vi "Contents Summary Text.vi"(11 "Message":refnum<class "VarMessage.lvclass">) -> (2 "Contents Summary Text":string, 3 "Message":refnum<class "VarMessage.lvclass">)   [LabVIEW 2011, in "Messenging.lvlib" / "VarMessage.lvclass"]
uses:
  VarMessage.lvclass
  <userlib>/_OpenG.lib/lvdata/lvdata.llb/Type Descriptor Enumeration__ogtk.ctl
  Send/Send.lvclass
  TextVarientMessage/MSG.lvclass
panel:
  out "Varient":variant
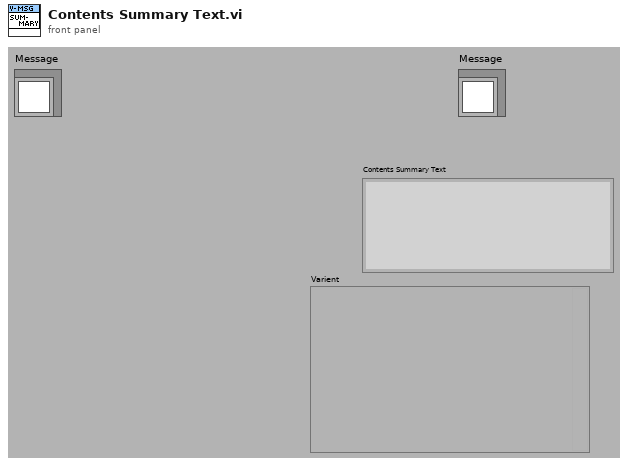
[diagram p1: front panel]
types:
  T1 = typedef "Type Descriptor Enumeration__ogtk.ctl" = enum8{"<Null>", "I8", "I16", "I32", "I64", "U8", "U16", "U32", "U64", "SGL", "DBL", "EXT", "CSG", "CDB", "CXT", "0x0F", "0x10", "0x11", "0x12", "0x13", "0x14", "Enum U8", "Enum U16", "Enum U32", "Enum U64", "SGL PQ", "DBL PQ", "EXT PQ", "CSG PQ", "CDB PQ", "CXT PQ", "0x1F", "0x20", "Boolean", "0x22", "0x23", "0x24", "0x25", "0x26", "0x27", "0x28", "0x29", "0x2A", "0x2B", "0x2C", "0x2D", "0x2E", "0x2F", "String", "0x31", "Path", "Pict", "0x34", "0x35", "0x36", "DAQ", "0x38", "0x39", "0x3A", "0x3B", "0x3C", "0x3D", "0x3E", "0x3F", "Array", "0x41", "0x42", "0x43", "0x44", "0x45", "0x46", "0x47", "0x48", "0x49", "0x4A", "0x4B", "0x4C", "0x4D", "0x4E", "0x4F", "Cluster", "0x51", "0x52", "Variant", "Waveform", "0x55", "0x56", "0x57", "0x58", "0x59", "0x5A", "0x5B", "0x5C", "0x5D", "0x5E", "0x5F", "0x60", "0x61", "0x62", "0x63", "0x64", "0x65", "0x66", "0x67", "0x68", "0x69", "0x6A", "0x6B", "0x6C", "0x6D", "0x6E", "0x6F", "Refnum"}
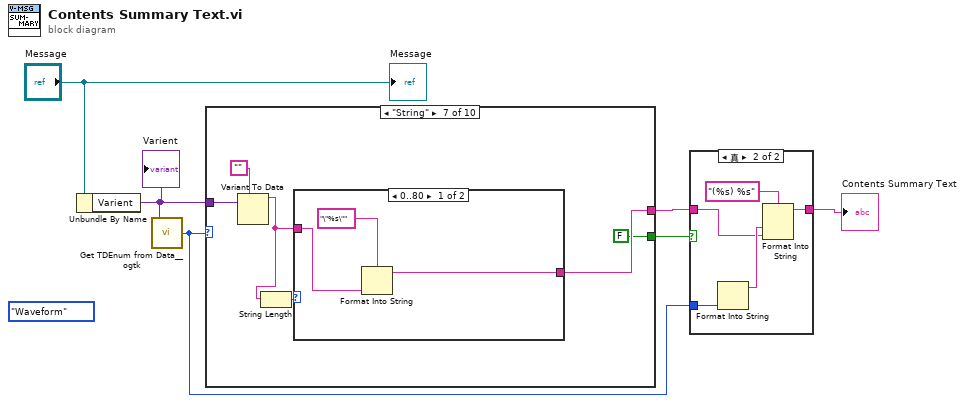
[diagram p0: block diagram]
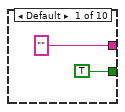
[diagram p3: hidden frame]
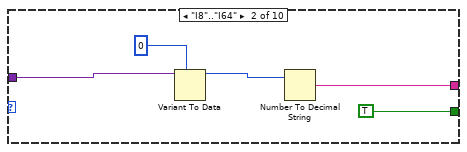
[diagram p4: hidden frame]
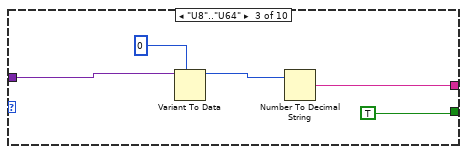
[diagram p5: hidden frame]
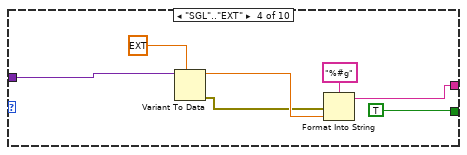
[diagram p6: hidden frame]
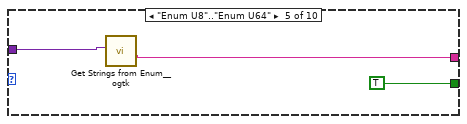
[diagram p7: hidden frame]
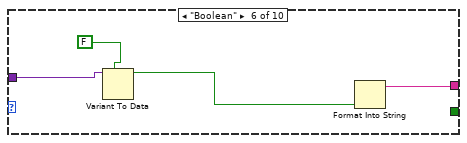
[diagram p8: hidden frame]
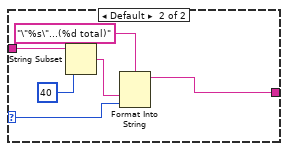
[diagram p9: hidden frame]
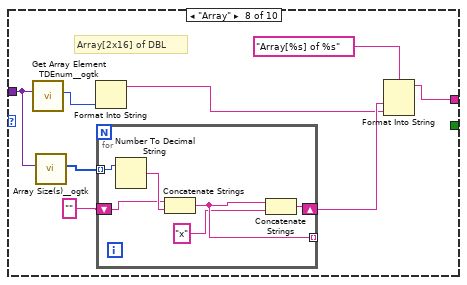
[diagram p10: hidden frame]
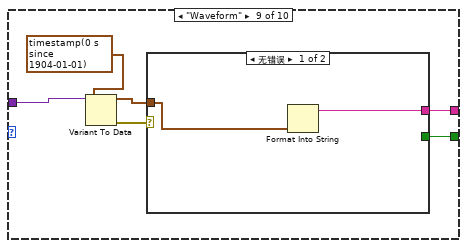
[diagram p11: hidden frame]
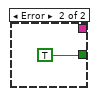
[diagram p12: hidden frame]
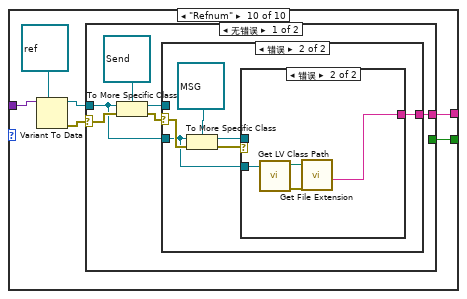
[diagram p13: hidden frame]
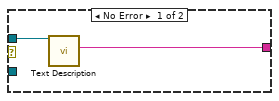
[diagram p14: hidden frame]
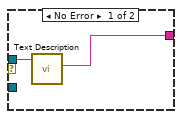
[diagram p15: hidden frame]
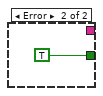
[diagram p16: hidden frame]
diagram:
  (unwired) Type_Descriptor_Enumeration__ogtk."Waveform" ("Type Descriptor Enumeration")
  n1 = Unbundle By Name("Message") -> ("Varient"=w1:variant)
  "Varient" <- w1
  n2 = call <userlib>:"Get TDEnum from Data__ogtk.vi"("Data"=w1) -> ("Type Descriptor Enumeration"=w5:T1)  [unwired: 4 out]
  n3 = case shown="\"String\"" w5 {
    tunnel: w1 -> [_ w13 w18 w25 w28 w31 w38 w54 w67 w76]
    tunnel: ["" w10 w15 w20 w26 w32 w34 w50 w63 w72] -> w3
    tunnel: [TRUE TRUE TRUE TRUE TRUE _ FALSE _ w62 w71] -> w2
    frame Default {
    }
    frame "I8".."I64" {
      n4 = Variant To Data(type=i64 0, Variant=w13) -> (data=w11:i64)  [unwired: 1 in, 1 out]
      n5 = Number To Decimal String(number=w11) -> (decimal integer string=w10:string)  [unwired: 1 out]
    }
    frame "U8".."U64" {
      n6 = Variant To Data(type=u64 0, Variant=w18) -> (data=w16:u64)  [unwired: 1 in, 1 out]
      n7 = Number To Decimal String(number=w16) -> (decimal integer string=w15:string)  [unwired: 1 out]
    }
    frame "SGL".."EXT" {
      n8 = Variant To Data(type=ext 0.0, Variant=w25) -> (data=w23:ext, error out=w22:errorcluster)  [unwired: 1 in]
      n9 = Format Into String(format string="%#g", error in=w22, w23) -> (resulting string=w20:string)  [unwired: 1 in, 1 out]
    }
    frame "Enum U8".."Enum U64" {
      n10 = call <userlib>:"Get Strings from Enum__ogtk.vi"("Enum"=w28) -> ("String Value"=w26:string)  [unwired: 1 in, 9 out]
    }
    frame "Boolean" {
      n11 = Variant To Data(type=FALSE, Variant=w31) -> (data=w29:bool)  [unwired: 1 in, 1 out]
      n12 = Format Into String(w29) -> (resulting string=w32:string)  [unwired: 3 in, 1 out]
    }
    frame "String" {
      n13 = Variant To Data(type="", Variant=w38) -> (data=w35:string)  [unwired: 1 in, 1 out]
      n14 = String Length(string=w35) -> (length=w36:i32)
      n15 = case shown="0..80" w36 {
        selector: w36 -> [_ w44]
        tunnel: w35 -> [w40 w47]
        tunnel: [w41 w43] -> w34
        frame 0..80 {
          n16 = Format Into String(format string="\"%s\"", w40) -> (resulting string=w41:string)  [unwired: 2 in, 1 out]
        }
        frame Default {
          n17 = String Subset(string=w47, length (rest)=40 ("length (rest)")) -> (substring=w42:string)  [unwired: 1 out]
          n18 = Format Into String(format string="\"%s\"...(%d total)", w42, w44) -> (resulting string=w43:string)  [unwired: 2 in, 1 out]
        }
      }
    }
    frame "Array" {
      # "Array[2x16] of DBL"
      n19 = call <userlib>:"Get Array Element TDEnum__ogtk.vi"("Array"=w54) -> ("Element Type"=w55:T1)  [unwired: 1 in, 9 out]
      n20 = call <userlib>:"Array Size(s)__ogtk.vi"("Array"=w54) -> ("Size(s)"=w53:u32[])  [unwired: 1 in, 9 out]
      n21 = Format Into String(w55) -> (resulting string=w48:string)  [unwired: 3 in, 1 out]
      n22 = for {
        tunnel: w53 -> [w61] mode=indexing
        shift-right: [w58] -> w49
        shift-left: "" -> [w59]
        tunnel: [w57] -> _ mode=indexing
        n23 = Number To Decimal String(number=w61) -> (decimal integer string=w60:string)  [unwired: 1 out]
        n24 = Concatenate Strings(w59, w60) -> (w57:string)
        n25 = Concatenate Strings(w57, "x") -> (w58:string)
      }
      n26 = Format Into String(format string="Array[%s] of %s", w49, w48) -> (resulting string=w50:string)  [unwired: 2 in, 1 out]
    }
    frame "Waveform" {
      n27 = Variant To Data(type=timestamp(0 s since 1904-01-01), Variant=w67) -> (data=w64:timestamp, error out=w65:errorcluster)  [unwired: 1 in]
      n28 = case shown="无错误" w65 {
        tunnel: w64 -> [w69 _]
        tunnel: [w68 _] -> w63
        tunnel: [_ TRUE] -> w62
        frame No Error {
          n29 = Format Into String(w69) -> (resulting string=w68:string)  [unwired: 3 in, 1 out]
        }
        frame Error {
        }
      }
    }
    frame "Refnum" {
      n30 = Variant To Data(type=refnum<class> refnum ("LabVIEW Object"), Variant=w76) -> (data=w73:refnum<class>, error out=w74:errorcluster)  [unwired: 1 in]
      n31 = case shown="无错误" w74 {
        selector: w74 -> [w78 _]
        tunnel: w73 -> [w77 _]
        tunnel: [w79 _] -> w72
        tunnel: [_ TRUE] -> w71
        frame No Error {
          n32 = To More Specific Class(target class=refnum<class "Send.lvclass"> refnum ("Messenging.lvlib:Send.lvclass"), reference=w77, error in=w78) -> (specific class reference=w80:refnum<class "Send.lvclass">, error out=w81:errorcluster)
          n33 = case shown="错误" w81 {
            selector: w81 -> [_ w90]
            tunnel: w80 -> [w84 _]
            tunnel: [w83 w86] -> w79
            tunnel: w77 -> [_ w85]
            frame No Error {
              n34 = call-dynamic "Text Description.vi"("Send in"=w84) -> ("Description"=w83:string)  [unwired: 10 out]
            }
            frame Error {
              n35 = To More Specific Class(target class=refnum<class "MSG.lvclass"> refnum ("Messenging.lvlib:Interprocess Message"), reference=w85, error in=w90) -> (specific class reference=w87:refnum<class "MSG.lvclass">, error out=w88:errorcluster)
              n36 = case shown="错误" w88 {
                tunnel: w87 -> [w92 _]
                tunnel: [w91 w93] -> w86
                tunnel: w85 -> [_ w96]
                frame No Error {
                  n37 = call-dynamic "Text Description.vi"("Message"=w92) -> ("Description"=w91:string)  [unwired: 10 out]
                }
                frame Error {
                  n38 = call <vilib>:"Get LV Class Path.vi"("object"=w96) -> ("error out"=w95:errorcluster, "class path"=w94:path)  [unwired: 1 in, 8 out]
                  n39 = call <vilib>:"Get File Extension.vi"("error in (no error)"=w95, "file"=w94) -> ("filename without extension"=w93:string)  [unwired: 9 out]
                }
              }
            }
          }
        }
        frame Error {
        }
      }
    }
  }
  n40 = case shown="真" w2 {
    tunnel: w5 -> [_ w103]
    tunnel: [w98 w102] -> w4
    tunnel: w3 -> [w98 w99]
    frame False {
    }
    frame True {
      n41 = Format Into String(w103) -> (resulting string=w101:string)  [unwired: 3 in, 1 out]
      n42 = Format Into String(format string="(%s) %s", w101, w99) -> (resulting string=w102:string)  [unwired: 2 in, 1 out]
    }
  }
  "Contents Summary Text" <- w4
  "Message" <- "Message"
